vi "hygro.vi"(0 "start":bool, 1 "temperatur":dbl, 3 "Fehlerkonstante":errorcluster) -> (6 "luftfeuchtigkeit":dbl, 7 "widerstand":dbl, 9 "Fehlerkonstante 2":errorcluster caption="Fehlerkonstante")   [LabVIEW 2013, in "TempHygro.lvlib"]
uses:
  lib/TempHygro.lvlib
  <vilib>/Analysis/5stat.llb/RMS (DBL).vi
  dll/libhygrometer.dll
  <vilib>/Analysis/NI_AALBase.lvlib
  <vilib>/Analysis/NI_AALPro.lvlib
panel:
  out "Waveform Graph":dbl[](graph)
  out "U_R1_RMS":dbl format="%0.2f"
  out "U_HYGRO_RMS":dbl
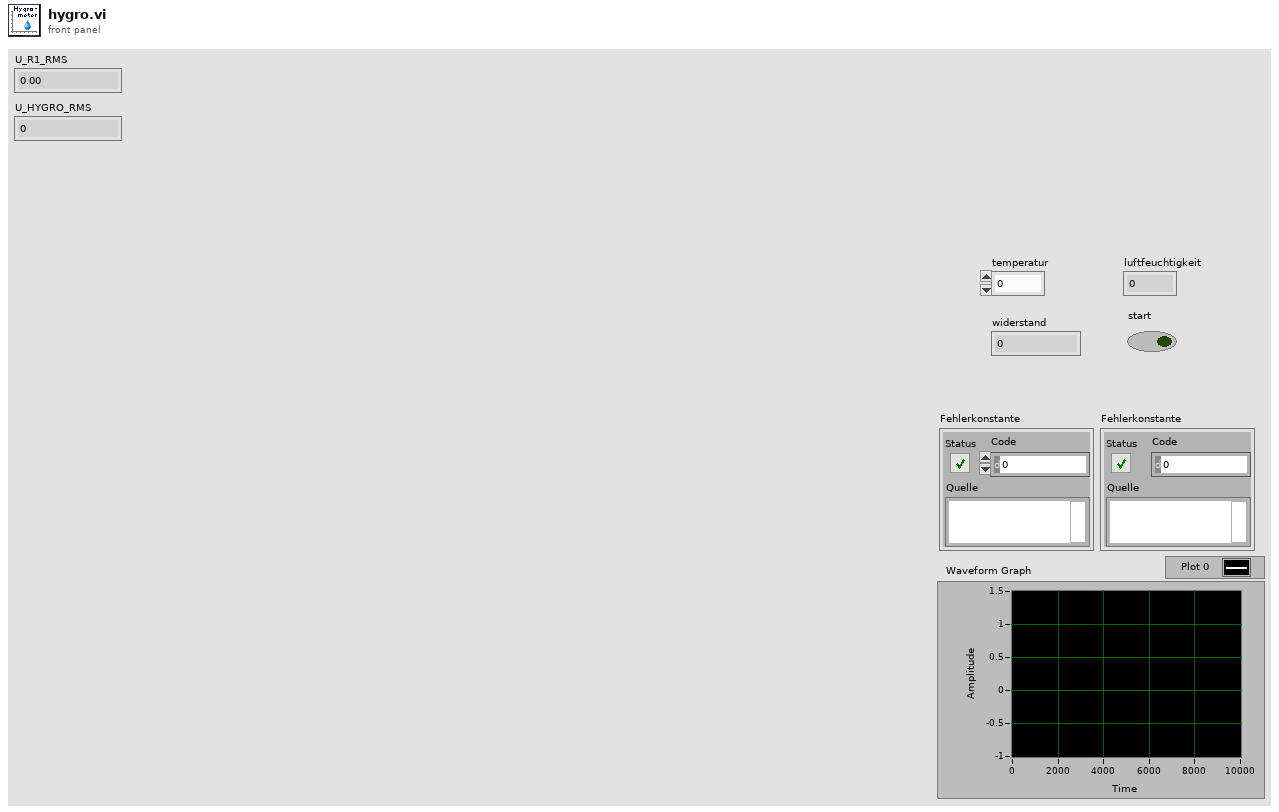
[diagram p1: front panel]
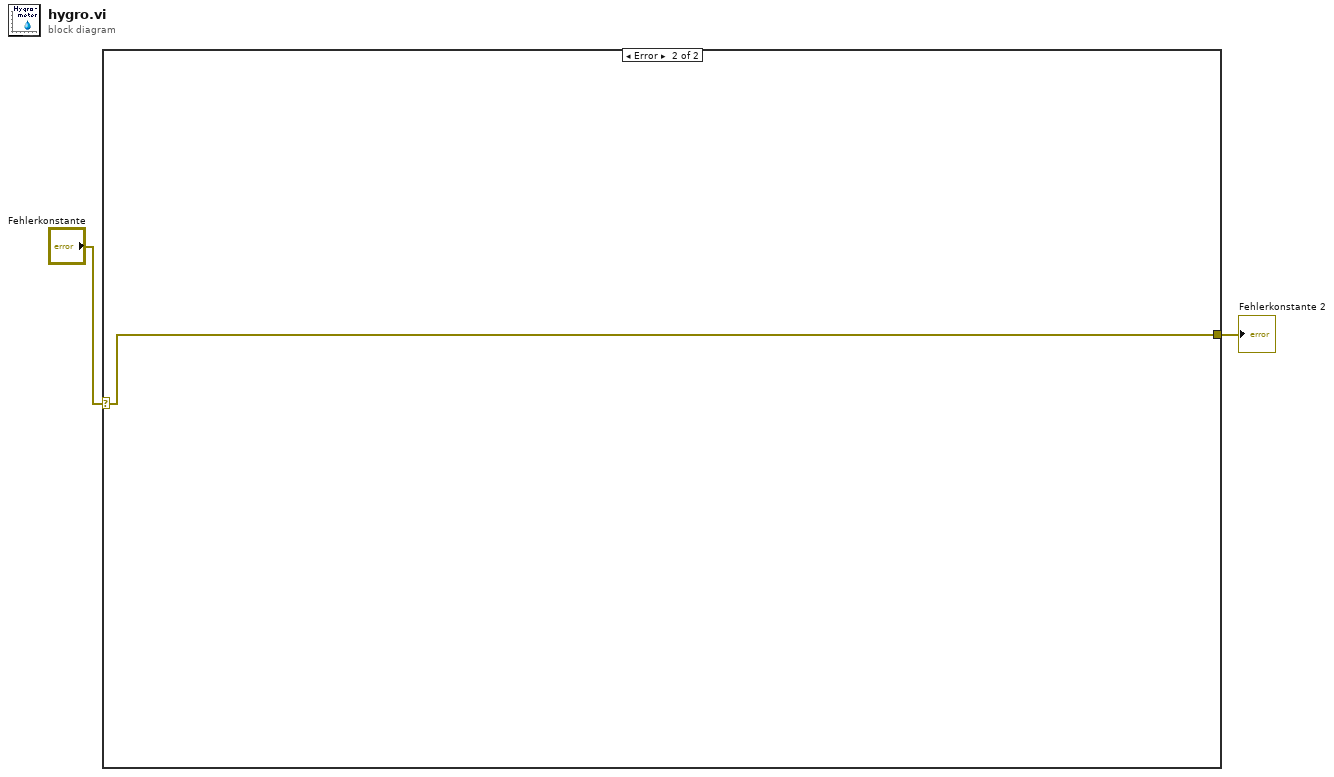
[diagram p0: block diagram]
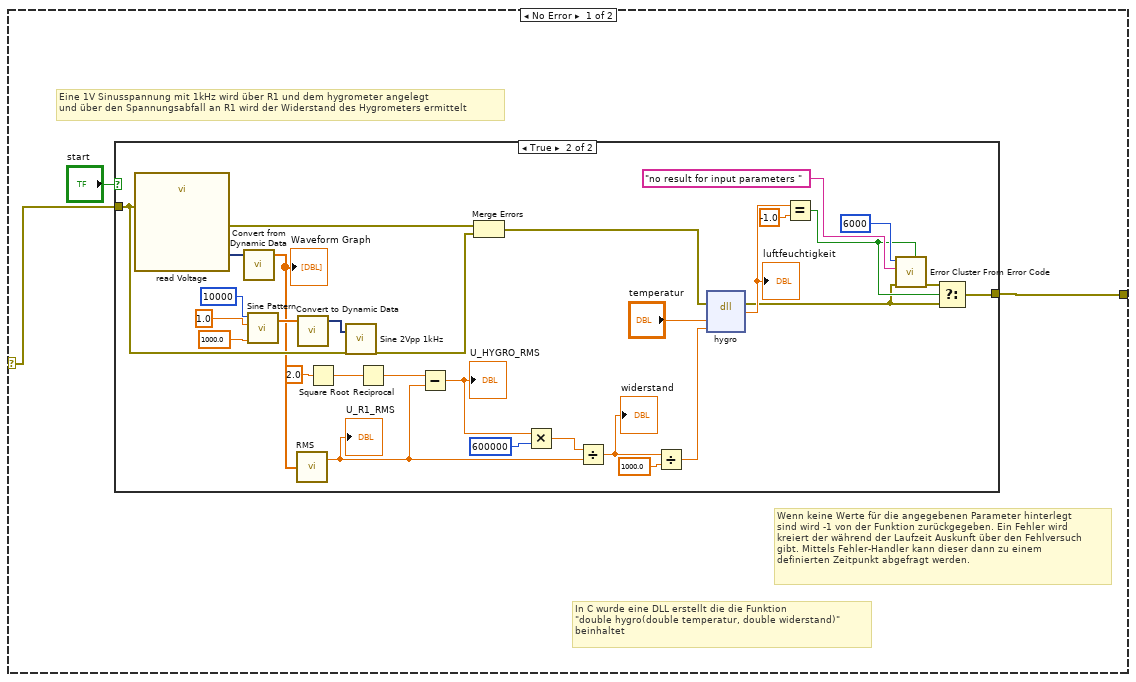
[diagram p2: hidden frame]
diagram:
  n1 = case shown="Error" "Fehlerkonstante" {
    selector: "Fehlerkonstante" -> [w3 w37]
    tunnel: [w4 w37] -> w2
    frame No Error {
      # "Eine 1V Sinusspannung mit 1kHz wird über R1 und dem hygrometer angelegt \nund über den Spannungsabfall an R1 wird der Widerstand des Hygrometers ermittelt"
      # "Wenn keine Werte für die angegebenen Parameter hinterlegt \nsind wird -1 von der Funktion zurückgegeben. Ein Fehler wird \nkreiert der während der Laufzeit Auskunft über den Fehlversuch\ngibt. Mittels Fehler-Handler kann dieser dann zu einem \ndefinierten Zeitpunkt abgefragt werden."
      # "In C wurde eine DLL erstellt die die Funktion \n\"double hygro(double temperatur, double widerstand)\" \nbeinhaltet"
      n2 = case shown="True" "start" {
        tunnel: w3 -> [w6 w16]
        tunnel: [w6 w9] -> w4
        frame False {
        }
        frame True {
          n3 = call "read Voltage"("error in"=w16) -> ("data"=w28:dynamicdata, "error out"=w20:errorcluster)  [unwired: 16 in, 1 out]
          n4 = call "Convert from Dynamic Data"("Dynamic Data Type"=w28) -> ("Array"=w13:dbl[])  [unwired: 3 in]
          "Waveform Graph" <- w13
          n5 = call <vilib>:"Sine Pattern.vi"("cycles"=1000.0, "amplitude"=1.0, "samples"=10000) -> ("Sinusoidal Pattern"=w17:dbl[])  [unwired: 1 in, 1 out]
          n6 = call-poly <vilib>:"RMS.vi"("X"=w13) -> ("rms value"=w24:dbl)  [unwired: 1 out]
          "U_R1_RMS" <- w24
          n7 = call "Convert to Dynamic Data"("Array"=w17) -> ("Dynamic Data Type"=w25:dynamicdata)  [unwired: 3 in]
          n8 = Square Root(x=2.0) -> (sqrt(x)=w23:dbl)
          n9 = call "Sine 2Vpp 1kHz"("data"=w25, "error in"=w16) -> ("error out"=w19:errorcluster)  [unwired: 16 in, 1 out]
          n10 = Reciprocal(x=w23) -> (1/x=w22:dbl)
          n11 = Subtract(x=w22, y=w24) -> (x-y=w31:dbl)
          "U_HYGRO_RMS" <- w31
          n12 = Merge Errors(w20, w19) -> (w15:errorcluster)
          n13 = Multiply(x=w31, y=600000) -> (x*y=w29:dbl)
          n14 = Divide(x=w29, y=w24) -> (x/y=w14:dbl)
          "widerstand" <- w14
          n15 = Divide(x=w14, y=1000.0) -> (x/y=w32:dbl)
          n16 = dll-call lib="C:/Users/waeis/Desktop/EMC-Program-master/res/dll/libhygrometer.dll" fn="hygro"(error in=w15, "temperatur"="temperatur", "widerstand"=w32) -> (error out=w7:errorcluster, "luftfeuchtigkeit"=w34:dbl)  [unwired: 4 in, 1 out]
          "luftfeuchtigkeit" <- w34
          n17 = Equal?(x=w34, y=-1.0) -> (x = y?=w10:bool)
          n18 = call <vilib>:"Error Cluster From Error Code.vi"("is warning? (False)"=w10, "error in (no error)"=w7, "error message (\"\")"="no result for input parameters " ("error message (\"\")"), "error code (0)"=6000) -> ("error out"=w8:errorcluster)  [unwired: 5 in]
          n19 = Select(t=w8, s=w10, f=w7) -> (s? t:f=w9:errorcluster)
        }
      }
    }
    frame Error {
    }
  }
  "Fehlerkonstante 2" <- w2
